vi "PCM_encode.vi"(8 "error in":errorcluster, 9 "Fs":dbl, 10 "voiceData":dbl[](array[numeric]), 11 "Path In":path) -> (0 "error out":errorcluster, 1 "encode_data":dbl[](array[numeric]), 2 "sampleData":dbl[](array[numeric]), 3 "Path Out":path)   [LabVIEW 2015]
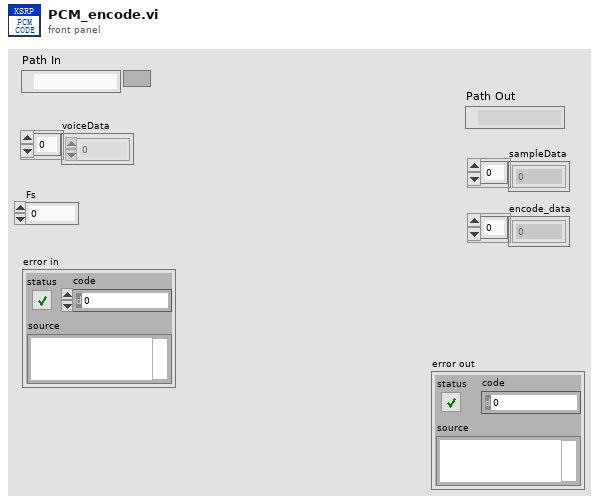
[diagram p1: front panel]
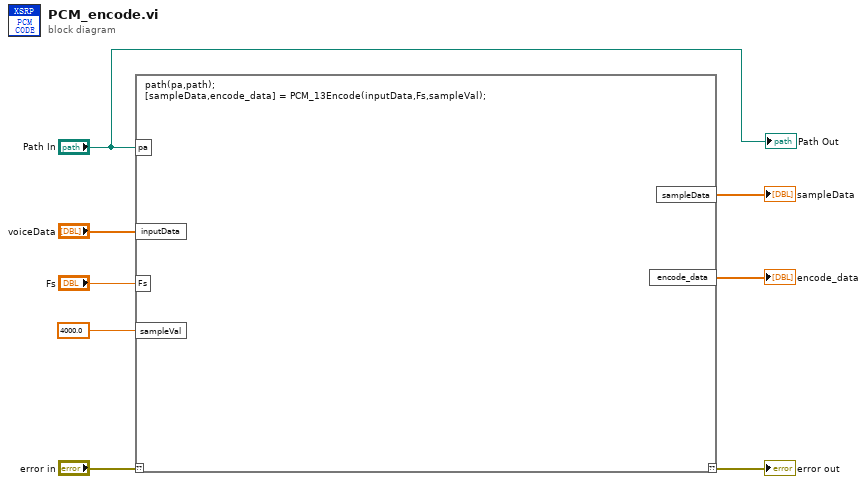
[diagram p0: block diagram]
diagram:
  n1 = script code="path(pa,path);\n[sampleData,encode_data] = PCM_13Encode(inputData,Fs,sampleVal);"("??"="error in", "pa"="Path In", "inputData"="voiceData", "Fs"="Fs", "sampleVal"=4000.0 ("sampelVal")) -> ("??"=→"error out":errorcluster, "sampleData"=→"sampleData":dbl[], "encode_data"=→"encode_data":dbl[])
  "Path Out" <- "Path In"
